vi "write column of data to json text.vi"(8 "error in":errorcluster, 9 "this vi path":path, 10 "column of data":string, 11 "file name":path) -> (0 "error out":errorcluster)   [LabVIEW 2020]
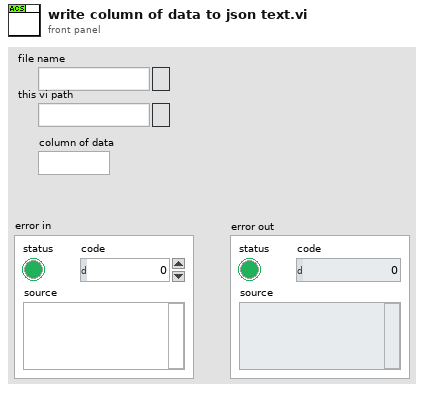
[diagram p1: front panel]
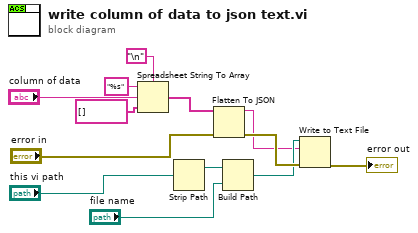
[diagram p0: block diagram]
diagram:
  n1 = Spreadsheet String To Array(delimiter (Tab)="\n", format string="%s", spreadsheet string="column of data", array type (2D Dbl)=string[] []) -> (array=w7:string[])
  n2 = Strip Path(path="this vi path") -> (stripped path=w8:path)  [unwired: 1 out]
  n3 = Flatten To JSON(anything=w7, error in (no error)="error in") -> (JSON string=w10:string, 11:w13:errorcluster)  [unwired: 1 in]
  n4 = Build Path(base path=w8, name or relative path="file name") -> (appended path=w12:path)
  n5 = Write to Text File(file (use dialog)=w12, text=w10, error in=w13) -> (error out=→"error out":errorcluster)  [unwired: 1 in, 2 out]
